vi "Get Tau.vi"(8 "error in":errorcluster, 10 "Data In":dbl[](array[numeric]), 11 "Fit Exp in":refnum<class "Fit Exponential.lvclass">) -> (0 "error out":errorcluster, 3 "Fit Exp out":refnum<class "Fit Exponential.lvclass">)   [LabVIEW 2014, in "Exponential Fit Library.lvlib" / "Fit Exponential.lvclass"]
doc: "This is the public method for the exponential strategy pattern."
uses:
  Fit Exponential.lvclass
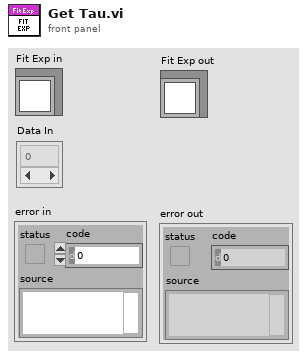
[diagram p1: front panel]
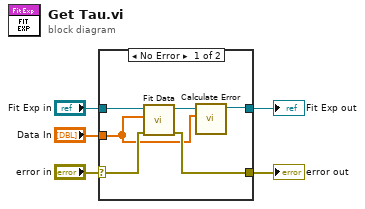
[diagram p0: block diagram]
diagram:
  n1 = case shown="No Error" "error in" {
    selector: "error in" -> [w9 w13]
    tunnel: [w8 w13] -> w4
    tunnel: [w7 w12] -> w2
    tunnel: "Fit Exp in" -> [w11 w12]
    tunnel: "Data In" -> [w6 _]
    frame No Error {
      n2 = call-dynamic "Fit Data.vi"("error in"=w9, "Data In"=w6, "Fit Exponential in"=w11) -> ("error out"=w8:errorcluster, "Fit Exponential out"=w10:refnum<class "Fit Exponential.lvclass">)  [unwired: 7 in]
      n3 = call "Calculate Error.vi"("X"=w6, "Fit Exp in"=w10) -> ("Fit Exp out"=w7:refnum<class "Fit Exponential.lvclass">)  [unwired: 9 in]
    }
    frame Error {
    }
  }
  "error out" <- w4
  "Fit Exp out" <- w2
